vi "Pre Loop Init.vi"(8 "error in (no error)":errorcluster, 11 "Ref In":refnum<vi>) -> (0 "error out":errorcluster, 3 "Event Registration Refnum":refnum<event-registration>)   [LabVIEW 2020, in "Error Handler.lvlib"]
uses:
  Error Handler.lvlib
  Private Controls/Element.ctl
  Private Controls/Module Action.ctl
  Queue FGV Action.ctl
  Architecture Support/Architecture Support.lvlib
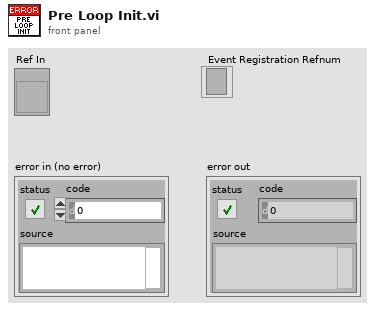
[diagram p1: front panel]
types:
  T1 = typedef "Error Handler.lvlib/Queue FGV Action.ctl" = enum16{"Get", "Set", "Release"}
  T2 = typedef "Error Handler.lvlib/Element.ctl" = cluster{"Action":T3, "Data":variant}
  T3 = typedef "Error Handler.lvlib/Module Action.ctl" = enum16{"Initialise Module", "Modify Reaction to Error", "Log to File", "Prompt User", "External Error", "Internal Error", "Exit"}
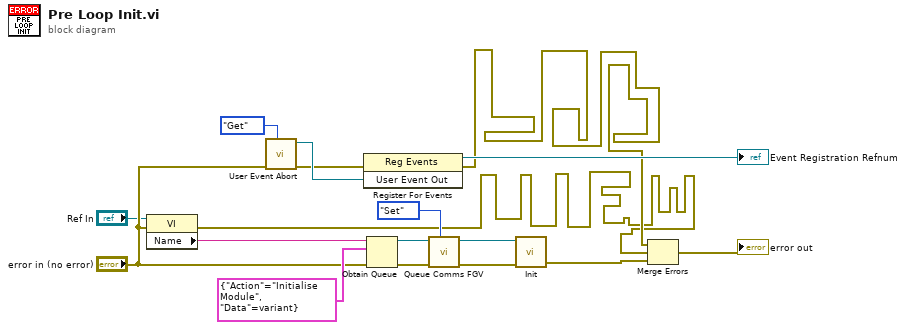
[diagram p0: block diagram]
diagram:
  n1 = property class="VI"(reference="Ref In", error in="error in (no error)") -> (error out=w1:errorcluster, "Name"=w12:string)  [unwired: 1 out]
  n2 = call "User Event Abort.vi"("Enum"=enum16{"Create", "Destroy", "Get"}."Get", "error in (no error)"="error in (no error)") -> ("error out"=w16:errorcluster, "User Event Out"=w17:refnum<user-event>)  [unwired: 8 in]
  n3 = register-events(error in=w16, w17) -> (reference out=→"Event Registration Refnum":refnum<event-registration>, error out=w2:errorcluster)  [unwired: 1 in]
  n4 = Obtain Queue(name (unnamed)=w12, element data type=T2 {"Action"=enum."Initialise Module", "Data"=variant} ("Element"), error in (no error)="error in (no error)") -> (queue out=w13:refnum<queue>, error out=w11:errorcluster)  [unwired: 2 in, 1 out]
  n5 = call "Queue Comms FGV.vi"("Action"=Queue_FGV_Action."Set", "error in (no error)"=w11, "queue In"=w13) -> ("error out"=w9:errorcluster, "queue In"=w8:refnum<queue>)  [unwired: 7 in]
  n6 = call "Init.vi"("error in (no error)"=w9, "Data"=w8) -> ("error out"=w5:errorcluster)  [unwired: 9 in]
  n7 = Merge Errors(w2, w1, w5) -> (→"error out":errorcluster)
